vi "Iteration Callback.vi"(7 "Owner":refnum<class>, 11 "Message":refnum<class "Message.lvclass">) -> (0 "error out":errorcluster)   [LabVIEW 2020]
uses:
  Message/Message.lvclass
  e7cc9b7e-b30c-4a73-b3cd-e343856a38b9.vi
  Message/Get Data.vi
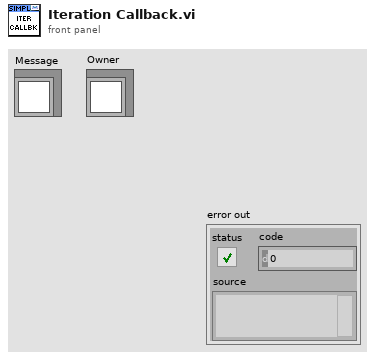
[diagram p1: front panel]
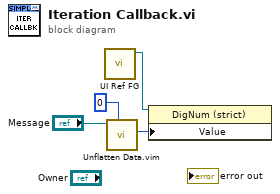
[diagram p0: block diagram]
diagram:
  n1 = call "UI Ref FG.vi"() -> ("Iteration"=w1:refnum<vi>)  [unwired: 9 in, 2 out]
  n2 = call "Unflatten Data.vim"("Data Type"=0, "Message in"="Message") -> ("Unflattened Data"=w4:i32)  [unwired: 7 in, 2 out]
  n3 = property class="DigNum (strict)"(reference=w1, "Value"=w4) -> ()  [unwired: 1 in, 2 out]
